vi "Ringdown_Display.vi"(0 "Data In":T4, 2 "Display State In":T2, 3 "Container State":T3) -> (6 "Data Out":T4, 7 "Display State Out":T2, 8 "Action":T1)   [LabVIEW 2015, in "Ringdown.xctl"]
uses:
  Ringdown.xctl
  Ringdown_Data.ctl
  <vilib>/_xctls/Container State.ctl
  Ringdown State.ctl
  <vilib>/_xctls/Action.ctl
  <vilib>/_xctls/XControlSupport.lvlib
panel:
  out "resGraph":sgl[][](graph)
  out "ringdown":sgl[][](graph)
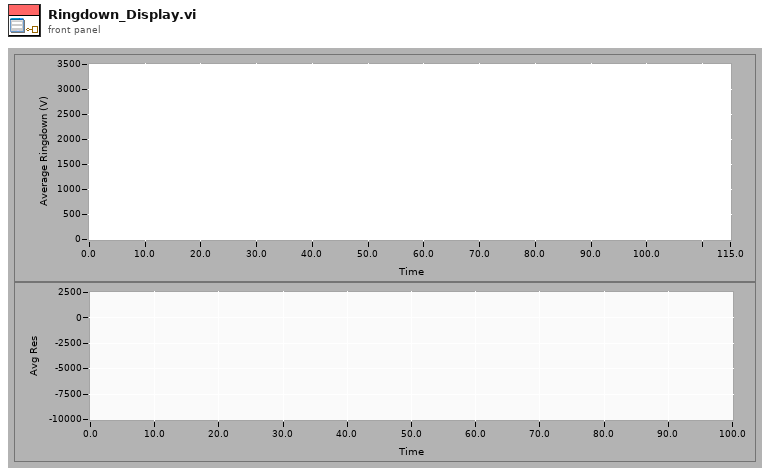
[diagram p1: front panel]
types:
  T1 = typedef "XControlSupport.lvlib/Action.ctl" = cluster{"Data Changed?":bool, "State Changed?":bool, "Action Name":string}
  T2 = typedef "Ringdown.xctl/Ringdown State.ctl" = cluster{"Dispaly Data":bool, "Display Fit":bool, "Trace":bool[], "RD Error ":bool, "Display Random":bool}
  T3 = typedef "XControlSupport.lvlib/Container State.ctl" = cluster{"Indicator?":bool, "Run Mode?":bool, " Refnum":refnum<vi>}
  T4 = typedef "Ringdown.xctl/Ringdown_Data.ctl" = i16[][][]
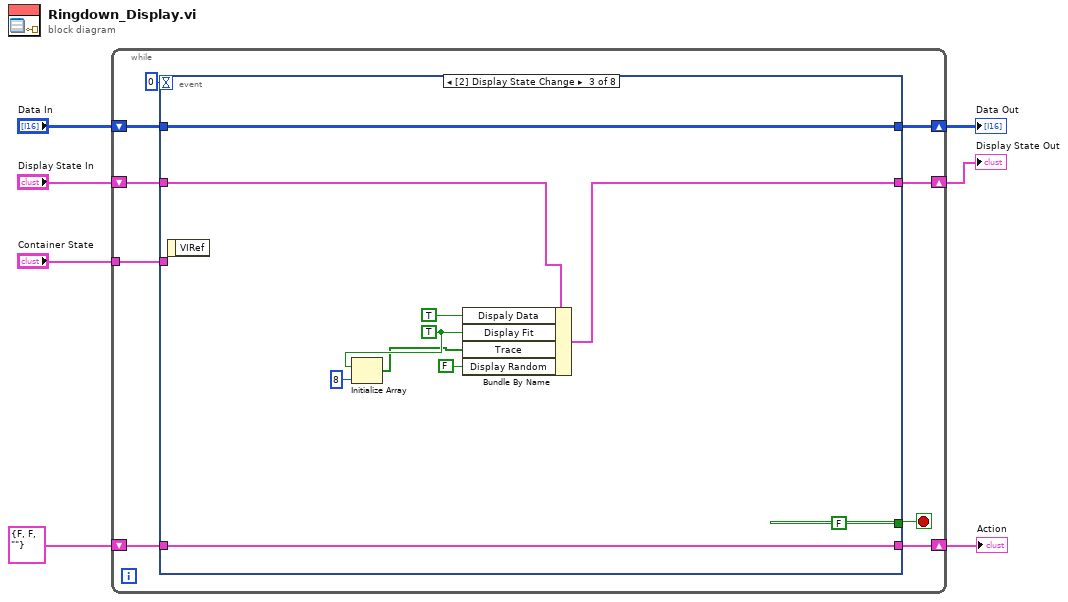
[diagram p0: block diagram]
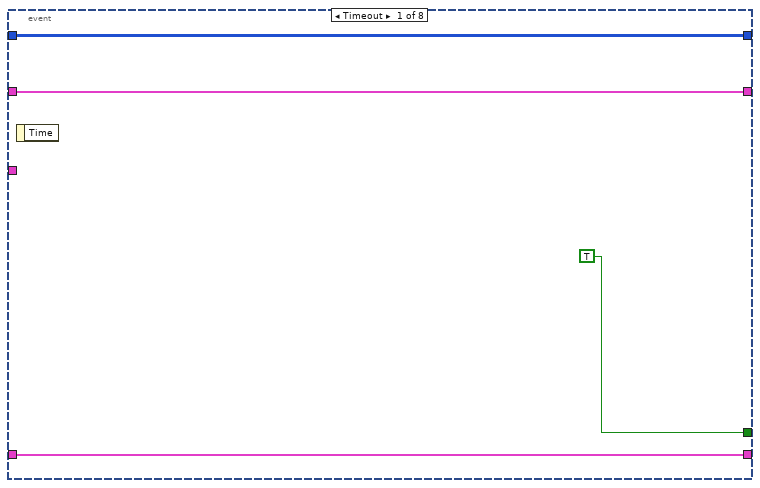
[diagram p2: hidden frame]
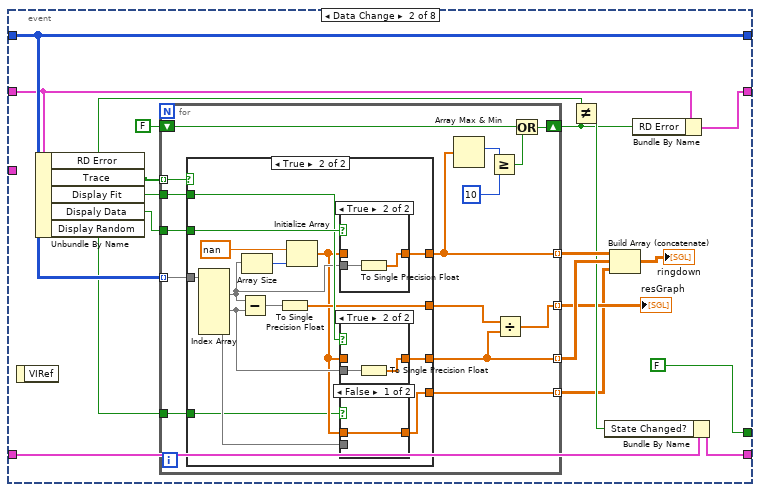
[diagram p3: hidden frame]
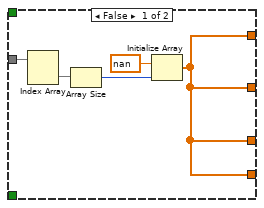
[diagram p4: hidden frame]
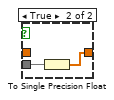
[diagram p5: hidden frame]
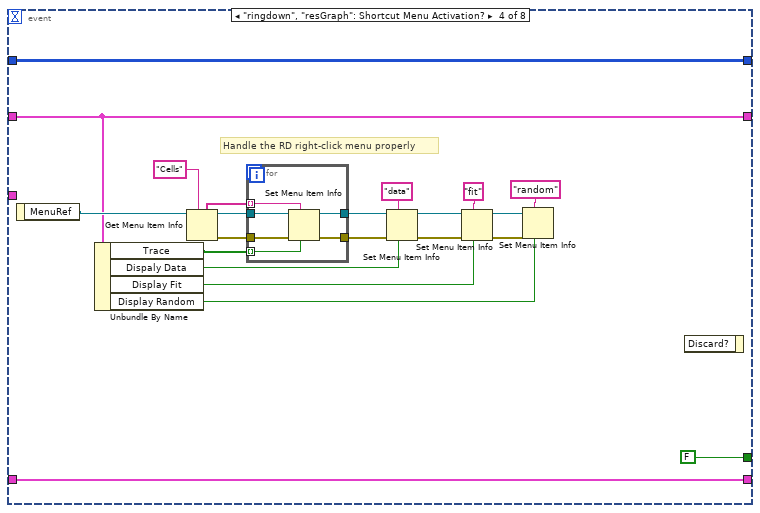
[diagram p8: hidden frame]
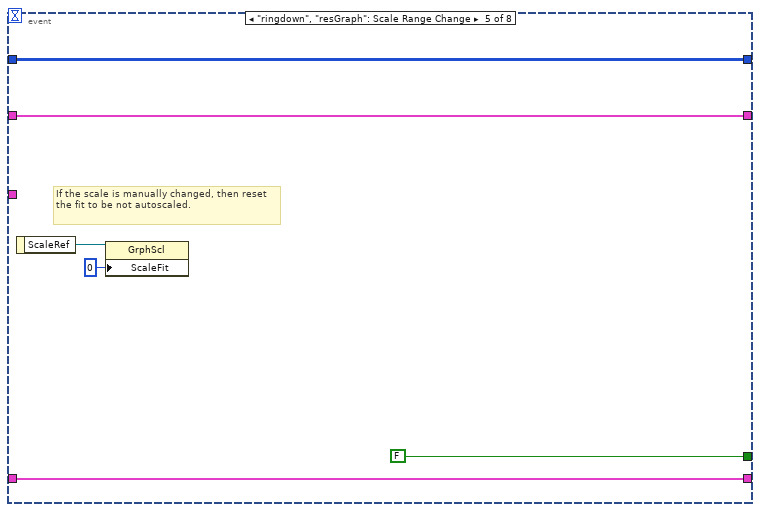
[diagram p9: hidden frame]
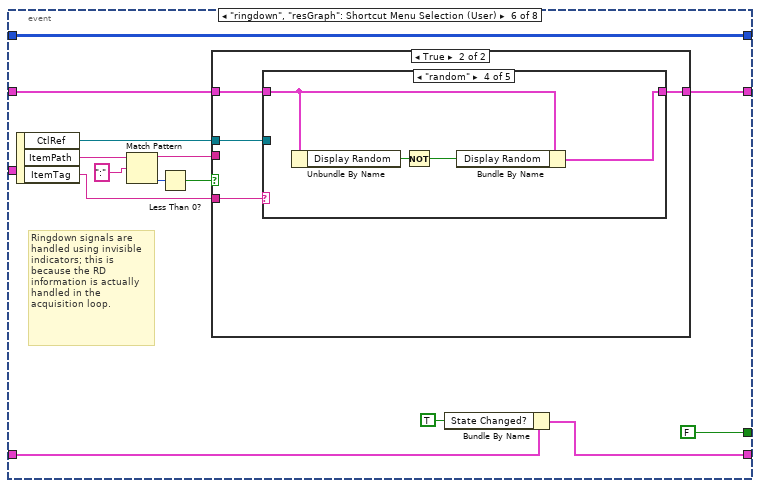
[diagram p10: hidden frame]
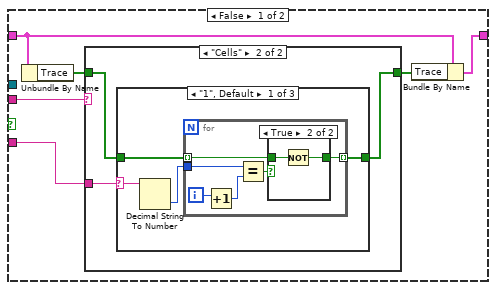
[diagram p11: hidden frame]
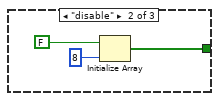
[diagram p14: hidden frame]
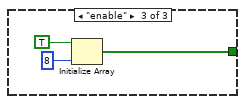
[diagram p15: hidden frame]
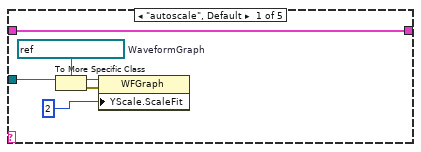
[diagram p16: hidden frame]
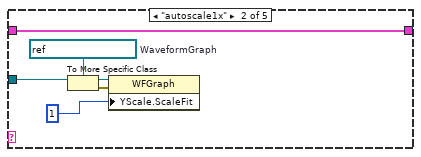
[diagram p17: hidden frame]
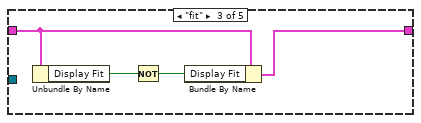
[diagram p18: hidden frame]
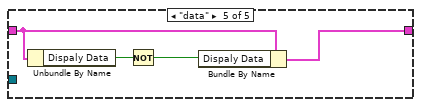
[diagram p19: hidden frame]
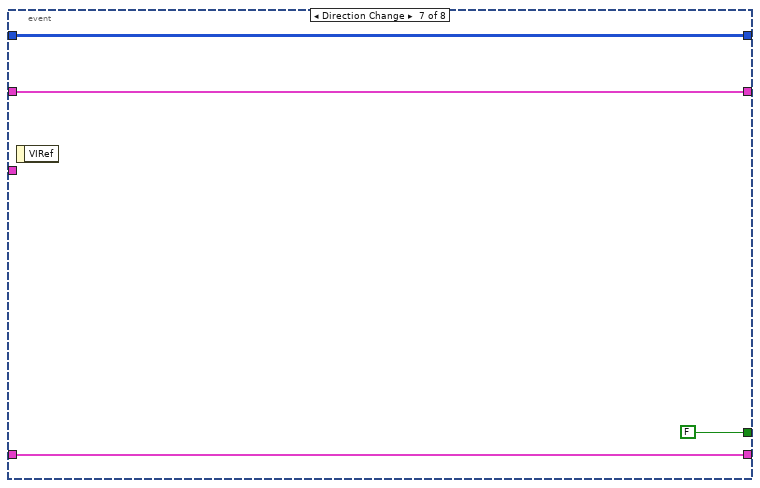
[diagram p20: hidden frame]
diagram:
  n1 = while {
    shift-right: [w15] -> w4
    shift-left: "Display State In" -> [w16]
    tunnel: "Container State" -> [w12]
    shift-right: [w10] -> w7
    shift-left: "Data In" -> [w11]
    shift-right: [w8] -> w2
    shift-left: T1 {"Data Changed?"=FALSE, "State Changed?"=FALSE, "Action Name"=""} ("Action") -> [w9]
    stop <- w14 stop-if-true
    n2 = event shown="[2] Display State Change" {
      selector: _ -> [_ _ _ _ _ _ _ _]
      dyn-events: _ -> [_ _ _ _ _ _ _ _]
      timeout: 0 -> [_ _ _ _ _ _ _ _]
      tunnel: w16 -> [w18 w27 w85 w102 w125 w131 w202 w209]
      tunnel: [w18 w26 w84 w102 w125 w130 w202 w203] -> w15
      tunnel: [TRUE FALSE FALSE FALSE FALSE FALSE FALSE FALSE] -> w14
      tunnel: w12 -> [_ _ _ _ _ _ _ _]
      tunnel: w11 -> [w17 w39 w93 w115 w124 w141 w201 w212]
      tunnel: [w17 w39 w93 w115 w124 w141 w201 w212] -> w10
      tunnel: [w19 w28 w92 w114 w123 w138 w200 w211] -> w8
      tunnel: w9 -> [w19 w30 w92 w114 w123 w140 w200 w211]
      event Timeout {
        n3 = event-data() -> ()  [unwired: 1 in, 1 out]
      }
      event Data Change {
        n4 = event-data() -> ()  [unwired: 1 in, 1 out]
        n5 = Unbundle By Name(w27) -> ("RD Error"=w31:bool, "Trace"=w38:bool[], "Display Fit"=w37:bool, "Dispaly Data"=w36:bool, "Display Random"=w21:bool)
        n6 = for {
          tunnel: w38 -> [w54] mode=indexing
          tunnel: [w45] -> w35 mode=indexing
          tunnel: [w43] -> w34 mode=indexing
          tunnel: [w42] -> w24 mode=indexing
          tunnel: w36 -> [w53]
          tunnel: w37 -> [w52]
          tunnel: w39 -> [w51] mode=indexing
          shift-right: [w46] -> w25
          shift-left: FALSE -> [w48]
          tunnel: [w41] -> w22 mode=indexing
          tunnel: w21 -> [w40]
          n7 = case shown="True" w54 {
            tunnel: [w55 w72] -> w45
            tunnel: [w55 w71] -> w43
            tunnel: [w55 w64] -> w44
            tunnel: w53 -> [_ w70]
            tunnel: w52 -> [_ w69]
            tunnel: w51 -> [w57 w68]
            tunnel: [w55 w60] -> w41
            tunnel: w40 -> [_ w61]
            frame False {
              n8 = Index Array(array=w57) -> (element=w56:i16[])  [unwired: 2 in]
              n9 = Array Size(array=w56) -> (size(s)=w59:i32)
              n10 = Initialize Array(sgl nan ("element"), w59) -> (w55:sgl[])
            }
            frame True {
              n11 = Index Array(array=w68) -> (element #1=w67:i16[], element #2=w66:i16[], element #3=w63:i16[])  [unwired: 6 in]
              n12 = Subtract(x=w67, y=w66) -> (x-y=w65:i16[])
              n13 = Array Size(array=w67) -> (size(s)=w73:i32)
              n14 = To Single Precision Float(number=w65) -> (single precision float=w64:sgl[])
              n15 = Initialize Array(sgl nan ("element"), w73) -> (w62:sgl[])
              n16 = case shown="True" w70 {
                tunnel: w62 -> [w81 _]
                tunnel: [w81 w82] -> w72
                tunnel: w67 -> [_ w83]
                frame False {
                }
                frame True {
                  n17 = To Single Precision Float(number=w83) -> (single precision float=w82:sgl[])
                }
              }
              n18 = case shown="True" w69 {
                tunnel: [w78 w79] -> w71
                tunnel: w66 -> [_ w80]
                tunnel: w62 -> [w78 _]
                frame False {
                }
                frame True {
                  n19 = To Single Precision Float(number=w80) -> (single precision float=w79:sgl[])
                }
              }
              n20 = case shown="False" w61 {
                tunnel: [w75 w76] -> w60
                tunnel: w63 -> [_ w77]
                tunnel: w62 -> [w75 _]
                frame False {
                }
                frame True {
                  n21 = To Single Precision Float(number=w77) -> (single precision float=w76:sgl[])
                }
              }
            }
          }
          n22 = Array Max & Min(array=w45) -> (max index (indices)=w50:i32)  [unwired: 3 out]
          n23 = Greater Or Equal?(x=w50, y=10) -> (x >= y?=w47:bool)
          n24 = Divide(x=w44, y=w43) -> (x/y=w42:sgl[])
          n25 = Or(x=w48, y=w47) -> (x .or. y?=w46:bool)
        }
        "resGraph" <- w24
        n26 = Not Equal?(x=w31, y=w25) -> (x != y?=w29:bool)
        n27 = Bundle By Name(cluster=w30, "State Changed?"=w29) -> (w28:T1)
        n28 = Build Array (concatenate)(w35, w34, w22) -> (→"ringdown":sgl[][])
        n29 = Bundle By Name(cluster=w27, "RD Error"=w25) -> (w26:T2)
      }
      event Display State Change {
        w88 = TRUE ("Display Fit")
        n30 = event-data() -> ()  [unwired: 1 in, 1 out]
        n31 = Initialize Array(w88, 8 ("dimension size")) -> (w86:bool[])
        n32 = Bundle By Name(cluster=w85, "Dispaly Data"=TRUE, "Display Fit"=w88, "Trace"=w86, "Display Random"=FALSE) -> (w84:T2)
      }
      event "ringdown", "resGraph": Shortcut Menu Activation? {
        # "Handle the RD right-click menu properly"
        n33 = event-data() -> ("MenuRef"=w103:refnum<k9>)  [unwired: 1 in]
        n34 = Unbundle By Name(w102) -> ("Trace"=w101:bool[], "Dispaly Data"=w99:bool, "Display Fit"=w100:bool, "Display Random"=w94:bool)
        n35 = Get Menu Item Info(7:"Cells" ("item tag"), 11:w103) -> (0:w106:errorcluster, 3:w112:refnum<k9>, 5:w111:string[])  [unwired: 1 in, 4 out]
        n36 = for {
          tunnel: w112 -> [w121]
          tunnel: w111 -> [w118] mode=indexing
          tunnel: w101 -> [w120] mode=indexing
          tunnel: [w119] -> w110
          tunnel: w106 -> [w117]
          tunnel: [w116] -> w105
          n37 = Set Menu Item Info(6:w120, 7:w118, 8:w117, 11:w121) -> (0:w116:errorcluster, 3:w119:refnum<k9>)  [unwired: 3 in]
        }
        n38 = Set Menu Item Info(6:w99, 7:"data" ("item tag"), 8:w105, 11:w110) -> (0:w104:errorcluster, 3:w108:refnum<k9>)  [unwired: 3 in]
        n39 = Set Menu Item Info(6:w100, 7:"fit" ("item tag"), 8:w104, 11:w108) -> (0:w95:errorcluster, 3:w96:refnum<k9>)  [unwired: 3 in]
        n40 = Set Menu Item Info(6:w94, 7:"random" ("item tag"), 8:w95, 11:w96) -> ()  [unwired: 3 in, 2 out]
        n41 = event-data() -> ()  [unwired: 2 in, 1 out]
      }
      event "ringdown", "resGraph": Scale Range Change {
        # "If the scale is manually changed, then reset the fit to be not autoscaled."
        n42 = event-data() -> ("ScaleRef"=w127:refnum<vi>)  [unwired: 1 in]
        n43 = property class="GrphScl"(reference=w127, "ScaleFit"=u8 0 ("Scale Fit")) -> ()  [unwired: 1 in, 2 out]
      }
      event "ringdown", "resGraph": Shortcut Menu Selection (User) {
        # "Ringdown signals are handled using invisible indicators; this is because the RD information is actually handled in the acquisition loop."
        n44 = event-data() -> ("CtlRef"=w129:refnum<vi>, "ItemPath"=w133:string, "ItemTag"=w132:string)  [unwired: 1 in]
        n45 = Match Pattern(string=w133, regular expression=":") -> (before substring=w134:string, offset past match=w136:i32)  [unwired: 1 in, 2 out]
        n46 = Less Than 0?(x=w136) -> (x < 0?=w135:bool)
        n47 = case shown="True" w135 {
          tunnel: w132 -> [w147 w174]
          tunnel: w134 -> [w146 _]
          tunnel: w131 -> [w144 w173]
          tunnel: [w142 w172] -> w130
          tunnel: w129 -> [_ w171]
          frame False {
            n48 = Unbundle By Name(w144) -> ("Trace"=w145:bool[])
            n49 = case shown="\"Cells\"" w146 {
              tunnel: w147 -> [_ w151]
              tunnel: w145 -> [w148 w150]
              tunnel: [w148 w149] -> w143
              frame "NULL", Default {
              }
              frame "Cells" {
                n50 = case shown="\"1\", Default" w151 {
                  selector: w151 -> [w155 _ _]
                  tunnel: [w153 w165 w168] -> w149
                  tunnel: w150 -> [w152 _ _]
                  frame "1", Default {
                    n51 = Decimal String To Number(string=w155) -> (number=w154:i32)  [unwired: 2 in, 1 out]
                    n52 = for {
                      tunnel: w152 -> [w159] mode=indexing
                      tunnel: w154 -> [w161]
                      tunnel: [w158] -> w153 mode=indexing
                      i -> [w157]
                      n53 = Increment(x=w157) -> (x+1=w156:i32)
                      n54 = Equal?(x=w161, y=w156) -> (x = y?=w160:bool)
                      n55 = case shown="True" w160 {
                        tunnel: w159 -> [w162 w164]
                        tunnel: [w162 w163] -> w158
                        frame False {
                        }
                        frame True {
                          n56 = Not(x=w164) -> (.not. x?=w163:bool)
                        }
                      }
                    }
                  }
                  frame "disable" {
                    n57 = Initialize Array(FALSE, 8 ("dimension size")) -> (w165:bool[])
                  }
                  frame "enable" {
                    n58 = Initialize Array(TRUE, 8 ("dimension size")) -> (w168:bool[])
                  }
                }
              }
            }
            n59 = Bundle By Name(cluster=w144, "Trace"=w143) -> (w142:T2)
          }
          frame True {
            n60 = case shown="\"random\"" w174 {
              tunnel: w173 -> [w179 w185 w190 w192 w197]
              tunnel: [w179 w185 w187 w191 w195] -> w172
              tunnel: w171 -> [w177 w183 _ _ _]
              frame "autoscale", Default {
                w178 = refnum<vi> refnum  # WaveformGraph
                n61 = To More Specific Class(target class=w178, reference=w177) -> (specific class reference=w176:refnum<vi>, error out=w175:errorcluster)  [unwired: 1 in]
                n62 = property on="Property Node" class="WFGraph"(reference=w176, error in=w175, "YScale.ScaleFit"=u8 2 ("Y Scale.Scale Fit")) -> ()  [unwired: 2 out]
              }
              frame "autoscale1x" {
                w184 = refnum<vi> refnum  # WaveformGraph
                n63 = To More Specific Class(target class=w184, reference=w183) -> (specific class reference=w182:refnum<vi>, error out=w181:errorcluster)  [unwired: 1 in]
                n64 = property on="Property Node" class="WFGraph"(reference=w182, error in=w181, "YScale.ScaleFit"=u8 1 ("Y Scale.Scale Fit")) -> ()  [unwired: 2 out]
              }
              frame "fit" {
                n65 = Unbundle By Name(w190) -> ("Display Fit"=w189:bool)
                n66 = Not(x=w189) -> (.not. x?=w188:bool)
                n67 = Bundle By Name(cluster=w190, "Display Fit"=w188) -> (w187:T2)
              }
              frame "random" {
                n68 = Unbundle By Name(w192) -> ("Display Random"=w194:bool)
                n69 = Not(x=w194) -> (.not. x?=w193:bool)
                n70 = Bundle By Name(cluster=w192, "Display Random"=w193) -> (w191:T2)
              }
              frame "data" {
                n71 = Unbundle By Name(w197) -> ("Dispaly Data"=w198:bool)
                n72 = Not(x=w198) -> (.not. x?=w196:bool)
                n73 = Bundle By Name(cluster=w197, "Dispaly Data"=w196) -> (w195:T2)
              }
            }
          }
        }
        n74 = Bundle By Name(cluster=w140, "State Changed?"=TRUE) -> (w138:T1)
      }
      event Direction Change {
        n75 = event-data() -> ()  [unwired: 1 in, 1 out]
      }
      event Exec State Change {
        w206 = TRUE ("Display Fit")
        n76 = event-data() -> ()  [unwired: 1 in, 1 out]
        n77 = Initialize Array(w206, 8 ("dimension size")) -> (w204:bool[])
        n78 = Bundle By Name(cluster=w209, "Dispaly Data"=TRUE, "Display Fit"=w206, "Trace"=w204, "Display Random"=FALSE) -> (w203:T2)
      }
    }
  }
  "Display State Out" <- w4
  "Data Out" <- w7
  "Action" <- w2
